vi "emballage affiche série en cours.vi"(1 "chaîne 2D":string) -> (0 "error out":errorcluster caption="sortie d'erreur")   [LabVIEW 2020]
doc: "Affiche les n° des pièces en cours d'emballage pour la commande en cours.\nSi une nouvelle commande est commencée, le tableau est remis à vide."
panel:
  in  "No pièce":string
  in  "quitter":bool
  out "Pièces en cours d'emballage":i32(listbox)
  # "Sélectionner\nl'élément"
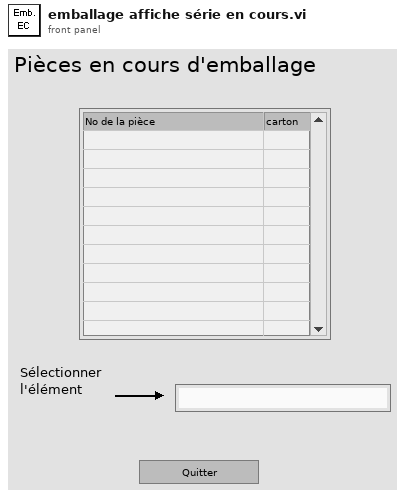
[diagram p1: front panel]
types:
  T1 = typedef "Emballage_BDD_param_Produit.ctl" = cluster{"No_Valve_FAS":string, "suffixe":string, "designation":string, "indice_produit":string, "code_barre_fixe":string, "affiche_code_barre_client":string, "affiche_no_client":string, "Nb_vlve_par_carton":u16, "melange_des_lots_possible":string, "id_article":string, "Indice_Rev":string, "Famille":string, "date":string, "code_barre_fixe_Fin":string, "Longeur_No_Serie":string}
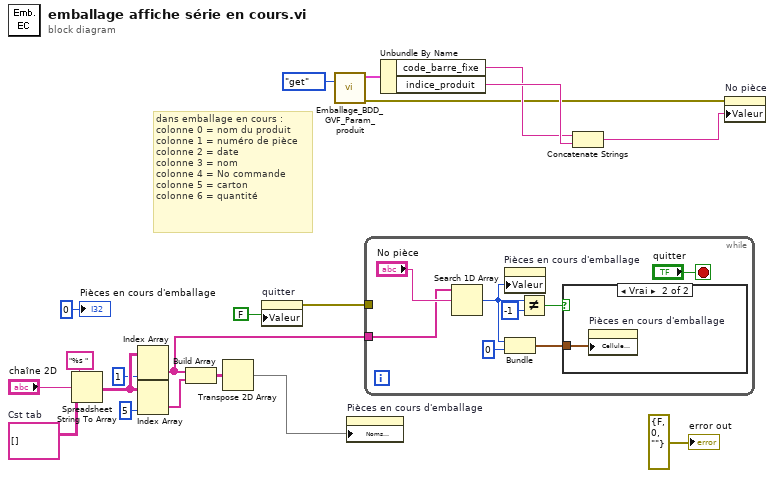
[diagram p0: block diagram]
diagram:
  w17 = string[][] []  # Cst tab
  # "dans emballage en cours :\ncolonne 0 = nom du produit\ncolonne 1 = numéro de pièce\ncolonne 2 = date\ncolonne 3 = nom\ncolonne 4 = No commande\ncolonne 5 = carton\ncolonne 6 = quantité"
  n1 = Spreadsheet String To Array(format string="%s ", spreadsheet string="chaîne 2D", array type (2D Dbl)=w17) -> (array=w16:string[][])  [unwired: 1 in]
  n2 = Index Array(array=w16, index (col)=1) -> (element=w11:string[])  [unwired: 1 in]
  n3 = Index Array(array=w16, index (col)=5) -> (element=w10:string[])  [unwired: 1 in]
  n4 = Build Array(w11, w10) -> (w9:string[][])
  n5 = Transpose 2D Array(2D array=w9) -> (transposed array=w8:string[][])
  n6 = property on="quitter" class="Bool (strict)"("Valeur"=FALSE) -> (error out=w19:errorcluster)  [unwired: 2 in, 1 out]
  n7 = call "Emballage_BDD_GVF_Param_produit.vi"("Énum"=enum16{"set", "get"}."get") -> ("Error out"=w2:errorcluster, "CLS_param_produit"=w4:T1)  [unwired: 7 in, 2 out]
  n8 = property on="Pièces en cours d'emballage" class="ListeMCol (strict)"("Noms d'éléments"=w8) -> ()  [unwired: 2 in, 2 out]
  n9 = while {
    tunnel: w19 -> [_]
    tunnel: w11 -> [w24]
    stop <- "quitter" stop-if-true
    n10 = Search 1D Array(1D array=w24, element="No pièce") -> (index of element=w23:i32)  [unwired: 1 in]
    n11 = property on="Pièces en cours d'emballage" class="ListeMCol (strict)"("Valeur"=w23) -> ()  [unwired: 2 in, 2 out]
    n12 = Bundle("index of element"=w23, 0) -> (w26:cluster{"index of element":i32, i32})  [unwired: 1 in]
    n13 = Not Equal?(x=w23, y=-1) -> (x != y?=w21:bool)
    n14 = case shown="Vrai" w21 {
      tunnel: w26 -> [_ w29]
      frame False {
      }
      frame True {
        n15 = property on="Pièces en cours d'emballage" class="ListeMCol (strict)"("Cellule visible en haut à gauche"=w29) -> ()  [unwired: 2 in, 2 out]
      }
    }
  }
  n16 = Unbundle By Name(w4) -> ("code_barre_fixe"=w5:string, "indice_produit"=w6:string)
  n17 = Concatenate Strings(w5, w6) -> (w3:string)
  n18 = property on="No pièce" class="Ch"(error in=w2, "Valeur"=w3) -> ()  [unwired: 1 in, 2 out]
  "Pièces en cours d'emballage" <- 0
  "error out" <- errorcluster {"status"=FALSE, "code"=0, "source"=""} ("error out")
